vi "Teleop.vi"(10 "Match Info":T1={"Autonomous Elapsed Seconds"=0.0, "TeleOp Elapsed Seconds"=0.0, "Disabled Elapsed Seconds"=0.0, "Visited Autonomous"=FALSE, "Visited TeleOp"=FALSE, "Visited Disabled"=FALSE, "Autonomous Settings"={"Autonomous Style"=enum."Independent", "VI Refnum"=refnum}}, 11 "Call Context":T2) -> ()   [LabVIEW 2017]
doc: "This VI is called for each enabled TeleOp packet received from the DS. It is typically used to read from joysticks and other inputs and update I/O or setpoints for timed control loops. It should complete and return within 20 milliseconds or risk missing DS packets."
uses:
  <vilib>/Rock Robotics/WPI/DriverStation/WPI_DriverStationDerivedRobotMode.ctl
  <vilib>/Rock Robotics/WPI/DriverStation/WPI_DriverStationMatch Info.ctl
  Framework/Robot Global Data.vi
panel:
  out "Hardware Fault":bool
  out "Temperature Fault":bool
  out "Battery Voltage Fault":bool
  out "Current Faults":bool[](array[boolean])
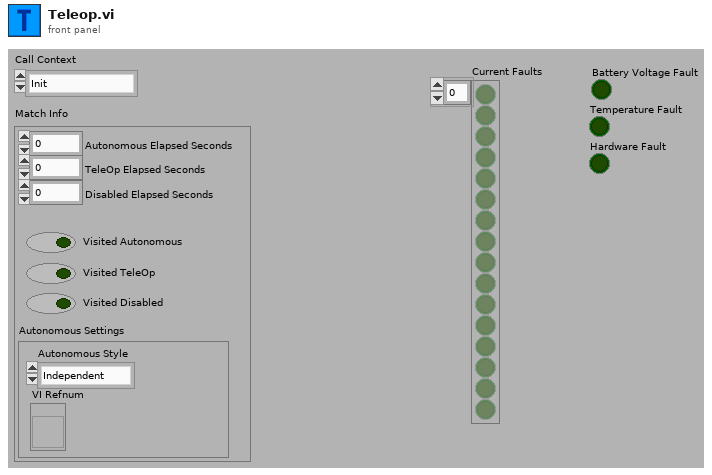
[diagram p1: front panel]
types:
  T1 = typedef "WPI_DriverStationMatch Info.ctl" = cluster{"Autonomous Elapsed Seconds":dbl, "TeleOp Elapsed Seconds":dbl, "Disabled Elapsed Seconds":dbl, "Visited Autonomous":bool, "Visited TeleOp":bool, "Visited Disabled":bool, "Autonomous Settings":cluster{"Autonomous Style":enum16{"Iterative", "Independent"}, "VI Refnum":refnum<vi>}}
  T2 = typedef "WPI_DriverStationDerivedRobotMode.ctl" = enum16{"Init", "Execute", "Stop"}
  T3 = enum16{"Linear", "Square  Root", "Square", "n^x"}
  T4 = enum16{"Normal", "Square", "Square with Rate", "Square Root", "Linear", "Exponential"}
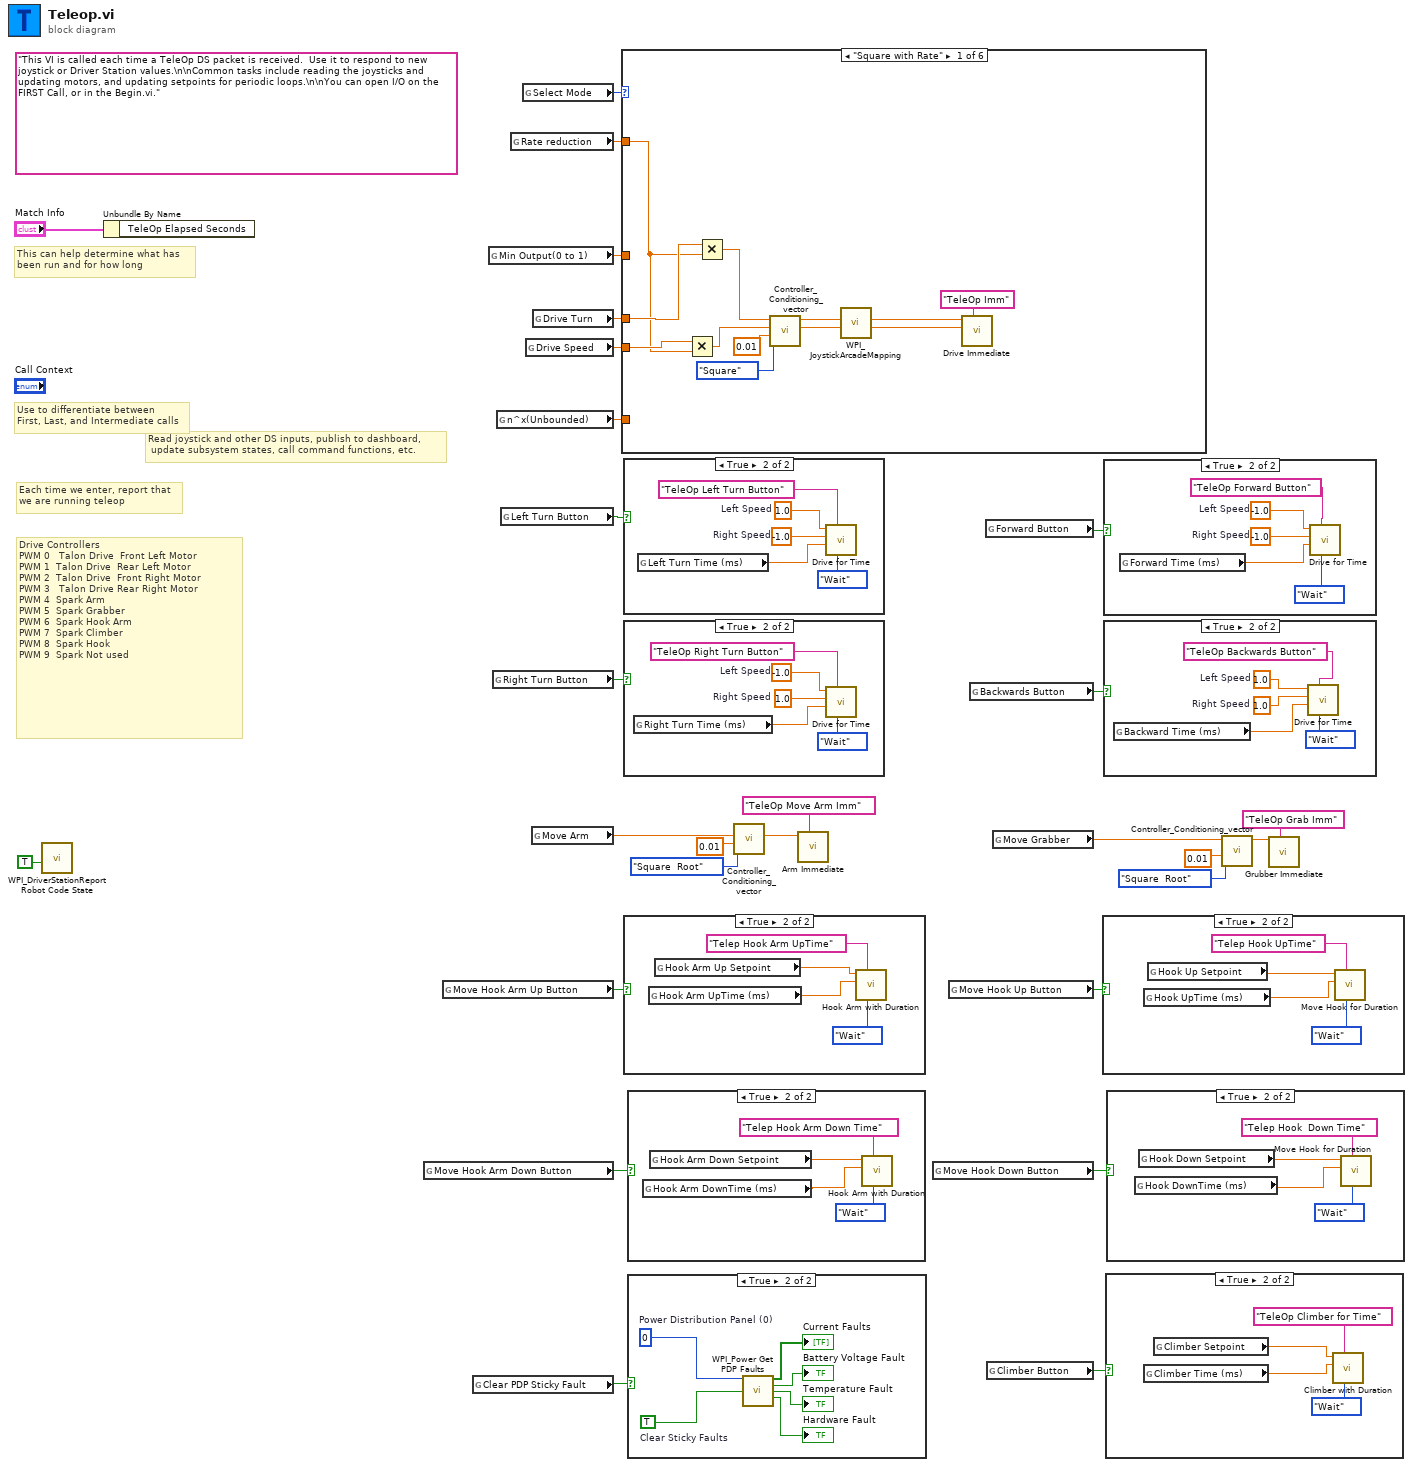
[diagram p0: block diagram]
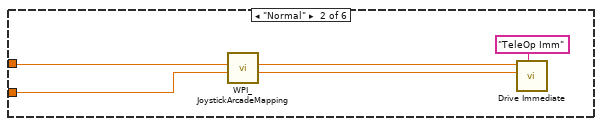
[diagram p12: hidden frame]
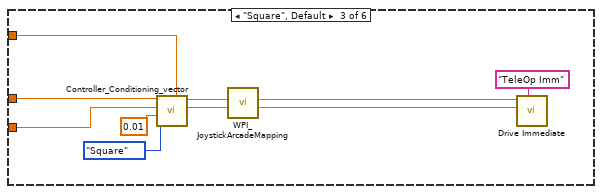
[diagram p13: hidden frame]
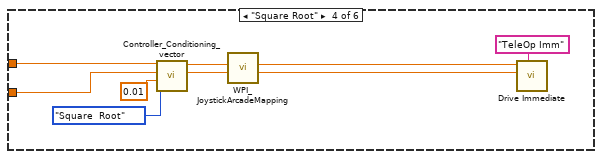
[diagram p14: hidden frame]
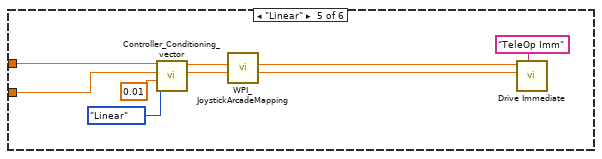
[diagram p15: hidden frame]
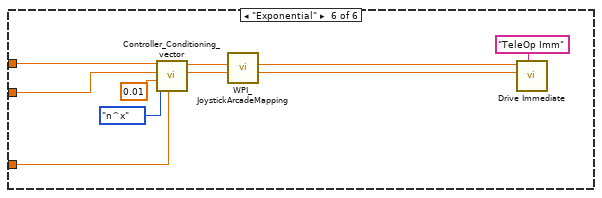
[diagram p16: hidden frame]
diagram:
  (unwired) "This VI is called each time a TeleOp DS packet is received.  Use it to respond to new joystick or Driver Station values.\n\nCommon tasks include reading the joysticks and updating motors, and updating setpoints for periodic loops.\n\nYou can open I/O on the FIRST Call, or in the Begin.vi."
  # "Drive Controllers\nPWM 0 \t\tTalon\tDrive \tFront Left Motor\nPWM 1\t\tTalon\tDrive \tRear Left Motor\nPWM 2\t\tTalon\tDrive \tFront Right Motor\nPWM 3 \t\tTalon\tDrive\tRear Right Motor\nPWM 4\t\tSpark\tArm\nPWM 5\t\tSpark\tGrabber\nPWM 6\t\tSpark\tHook Arm\nPWM 7\t\tSpark\tClimber\nPWM 8\t\tSpark\tHook\nPWM 9\t\tSpark\tNot used"
  # "Read joystick and other DS inputs, publish to dashboard,\n update subsystem states, call command functions, etc."
  # "Each time we enter, report that\nwe are running teleop"
  # "Use to differentiate between\nFirst, Last, and Intermediate calls"
  # "This can help determine what has\nbeen run and for how long"
  n1 = call <vilib>:"WPI_DriverStationReport Robot Code State.vi"("TeleOp"=TRUE ("Autonomous")) -> ()  [unwired: 10 in, 1 out]
  n2 = Unbundle By Name("Match Info") -> ()  [unwired: 1 out]
  n3 = global read "Robot Global Data.vi" "Move Hook Arm Down Button"() -> (w14:bool)
  n4 = global read "Robot Global Data.vi" "Move Hook Arm Up Button"() -> (w15:bool)
  n5 = global read "Robot Global Data.vi" "Clear PDP Sticky Fault"() -> (w16:bool)
  n6 = global read "Robot Global Data.vi" "Min Output(0 to 1)"() -> (w25:dbl)
  n7 = global read "Robot Global Data.vi" "Right Turn Button"() -> (w19:bool)
  n8 = global read "Robot Global Data.vi" "n^x(Unbounded)"() -> (w24:dbl)
  n9 = global read "Robot Global Data.vi" "Left Turn Button"() -> (w20:bool)
  n10 = global read "Robot Global Data.vi" "Rate reduction"() -> (w23:dbl)
  n11 = global read "Robot Global Data.vi" "Select Mode"() -> (w26:T4)
  n12 = global read "Robot Global Data.vi" "Drive Speed"() -> (w21:dbl)
  n13 = global read "Robot Global Data.vi" "Move Arm"() -> (w18:dbl)
  n14 = global read "Robot Global Data.vi" "Drive Turn"() -> (w22:dbl)
  n15 = case shown="\"Square with Rate\"" w26 {
    tunnel: w22 -> [w40 w42 w47 w56 w65 w75]
    tunnel: w21 -> [w39 w41 w48 w57 w66 w76]
    tunnel: w25 -> [_ _ w46 _ _ _]
    tunnel: w24 -> [_ _ _ _ _ w74]
    tunnel: w23 -> [w29 _ _ _ _ _]
    frame "Square with Rate" {
      n16 = Multiply(x=w39, y=w29) -> (x*y=w30:dbl)
      n17 = Multiply(x=w40, y=w29) -> (x*y=w31:dbl)
      n18 = call "Controller_Conditioning_vector.vi"("Enum"=T3."Square", "Dead Zone(0 to 1)"=0.01, "Y(-1 to 1)"=w30, "X(-1 to 1)"=w31) -> ("Y"=w32:dbl, "X"=w33:dbl)  [unwired: 4 in, 2 out]
      n19 = call <vilib>:"WPI_JoystickArcadeMapping.vi"("Y axis value"=w32, "X axis value"=w33) -> ("Right Motor Value"=w36:dbl, "Left Motor Value"=w37:dbl)  [unwired: 8 in]
      n20 = call "Drive Immediate.vi"("Description"="TeleOp Imm", "Right Setpoint"=w36, "Left Setpoint"=w37) -> ()  [unwired: 8 in, 1 out]
    }
    frame "Normal" {
      n21 = call <vilib>:"WPI_JoystickArcadeMapping.vi"("Y axis value"=w41, "X axis value"=w42) -> ("Right Motor Value"=w43:dbl, "Left Motor Value"=w44:dbl)  [unwired: 8 in]
      n22 = call "Drive Immediate.vi"("Description"="TeleOp Imm", "Right Setpoint"=w43, "Left Setpoint"=w44) -> ()  [unwired: 8 in, 1 out]
    }
    frame "Square", Default {
      n23 = call "Controller_Conditioning_vector.vi"("Min Output(0 to 1)"=w46, "Enum"=T3."Square", "Dead Zone(0 to 1)"=0.01, "Y(-1 to 1)"=w48, "X(-1 to 1)"=w47) -> ("Y"=w49:dbl, "X"=w50:dbl)  [unwired: 3 in, 2 out]
      n24 = call <vilib>:"WPI_JoystickArcadeMapping.vi"("Y axis value"=w49, "X axis value"=w50) -> ("Right Motor Value"=w53:dbl, "Left Motor Value"=w54:dbl)  [unwired: 8 in]
      n25 = call "Drive Immediate.vi"("Description"="TeleOp Imm", "Right Setpoint"=w53, "Left Setpoint"=w54) -> ()  [unwired: 8 in, 1 out]
    }
    frame "Square Root" {
      n26 = call "Controller_Conditioning_vector.vi"("Enum"=T3."Square  Root", "Dead Zone(0 to 1)"=0.01, "Y(-1 to 1)"=w57, "X(-1 to 1)"=w56) -> ("Y"=w58:dbl, "X"=w59:dbl)  [unwired: 4 in, 2 out]
      n27 = call <vilib>:"WPI_JoystickArcadeMapping.vi"("Y axis value"=w58, "X axis value"=w59) -> ("Right Motor Value"=w62:dbl, "Left Motor Value"=w63:dbl)  [unwired: 8 in]
      n28 = call "Drive Immediate.vi"("Description"="TeleOp Imm", "Right Setpoint"=w62, "Left Setpoint"=w63) -> ()  [unwired: 8 in, 1 out]
    }
    frame "Linear" {
      n29 = call "Controller_Conditioning_vector.vi"("Enum"=T3."Linear", "Dead Zone(0 to 1)"=0.01, "Y(-1 to 1)"=w66, "X(-1 to 1)"=w65) -> ("Y"=w67:dbl, "X"=w68:dbl)  [unwired: 4 in, 2 out]
      n30 = call <vilib>:"WPI_JoystickArcadeMapping.vi"("Y axis value"=w67, "X axis value"=w68) -> ("Right Motor Value"=w71:dbl, "Left Motor Value"=w72:dbl)  [unwired: 8 in]
      n31 = call "Drive Immediate.vi"("Description"="TeleOp Imm", "Right Setpoint"=w71, "Left Setpoint"=w72) -> ()  [unwired: 8 in, 1 out]
    }
    frame "Exponential" {
      n32 = call "Controller_Conditioning_vector.vi"("n^x(Unbounded)"=w74, "Enum"=T3."n^x", "Dead Zone(0 to 1)"=0.01, "Y(-1 to 1)"=w76, "X(-1 to 1)"=w75) -> ("Y"=w77:dbl, "X"=w78:dbl)  [unwired: 3 in, 2 out]
      n33 = call <vilib>:"WPI_JoystickArcadeMapping.vi"("Y axis value"=w77, "X axis value"=w78) -> ("Right Motor Value"=w81:dbl, "Left Motor Value"=w82:dbl)  [unwired: 8 in]
      n34 = call "Drive Immediate.vi"("Description"="TeleOp Imm", "Right Setpoint"=w81, "Left Setpoint"=w82) -> ()  [unwired: 8 in, 1 out]
    }
  }
  n35 = case shown="True" w20 {
    frame False {
    }
    frame True {
      w86 = -1.0  # Right Speed
      w85 = 1.0  # Left Speed
      n36 = global read "Robot Global Data.vi" "Left Turn Time (ms)"() -> (w84:dbl)
      n37 = call "Drive for Time.vi"("Synchronization"=enum16{"Start", "Wait"}."Wait" ("Synchronication"), "Description"="TeleOp Left Turn Button", "Duration (ms)"=w84, "Right Speed"=w86, "Left Speed"=w85) -> ()  [unwired: 5 in, 2 out]
    }
  }
  n38 = case shown="True" w19 {
    frame False {
    }
    frame True {
      w91 = 1.0  # Right Speed
      w90 = -1.0  # Left Speed
      n39 = global read "Robot Global Data.vi" "Right Turn Time (ms)"() -> (w89:dbl)
      n40 = call "Drive for Time.vi"("Synchronization"=enum16{"Start", "Wait"}."Wait" ("Synchronication"), "Description"="TeleOp Right Turn Button", "Duration (ms)"=w89, "Right Speed"=w91, "Left Speed"=w90) -> ()  [unwired: 5 in, 2 out]
    }
  }
  n41 = case shown="True" w15 {
    frame False {
    }
    frame True {
      n42 = global read "Robot Global Data.vi" "Hook Arm UpTime (ms)"() -> (w95:dbl)
      n43 = global read "Robot Global Data.vi" "Hook Arm Up Setpoint"() -> (w94:dbl)
      n44 = call "Hook Arm with Duration.vi"("Synchronization"=enum16{"Start", "Wait"}."Wait", "Description"="Telep Hook Arm UpTime", "Duration (ms)"=w95, "Setpoint"=w94) -> ()  [unwired: 7 in, 1 out]
    }
  }
  n45 = case shown="True" w14 {
    frame False {
    }
    frame True {
      n46 = global read "Robot Global Data.vi" "Hook Arm DownTime (ms)"() -> (w99:dbl)
      n47 = global read "Robot Global Data.vi" "Hook Arm Down Setpoint"() -> (w98:dbl)
      n48 = call "Hook Arm with Duration.vi"("Synchronization"=enum16{"Start", "Wait"}."Wait", "Description"="Telep Hook Arm Down Time", "Duration (ms)"=w99, "Setpoint"=w98) -> ()  [unwired: 7 in, 1 out]
    }
  }
  n49 = case shown="True" w16 {
    frame False {
    }
    frame True {
      w106 = TRUE  # Clear Sticky Faults
      w107 = u8 0  # Power Distribution Panel (0)
      n50 = call <vilib>:"WPI_Power Get PDP Faults.vi"("Power Distribution Panel (0)"=w107, "Clear Sticky Faults"=w106) -> ("Current Faults"=→"Current Faults":bool[], "Battery Voltage Fault"=→"Battery Voltage Fault":bool, "Temperature Fault"=→"Temperature Fault":bool, "Hardware Fault"=→"Hardware Fault":bool)  [unwired: 9 in, 1 out]
    }
  }
  n51 = call "Controller_Conditioning_vector.vi"("Enum"=T3."Square  Root", "Dead Zone(0 to 1)"=0.01, "Y(-1 to 1)"=w18) -> ("Y"=w9:dbl)  [unwired: 5 in, 3 out]
  n52 = call "Arm Immediate.vi"("Description"="TeleOp Move Arm Imm", "Setpoint"=w9) -> ()  [unwired: 9 in, 1 out]
  n53 = global read "Robot Global Data.vi" "Move Hook Down Button"() -> (w3:bool)
  n54 = global read "Robot Global Data.vi" "Move Hook Up Button"() -> (w2:bool)
  n55 = global read "Robot Global Data.vi" "Backwards Button"() -> (w13:bool)
  n56 = global read "Robot Global Data.vi" "Forward Button"() -> (w12:bool)
  n57 = global read "Robot Global Data.vi" "Climber Button"() -> (w1:bool)
  n58 = global read "Robot Global Data.vi" "Move Grabber"() -> (w17:dbl)
  n59 = case shown="True" w2 {
    frame False {
    }
    frame True {
      n60 = global read "Robot Global Data.vi" "Hook UpTime (ms)"() -> (w109:dbl)
      n61 = global read "Robot Global Data.vi" "Hook Up Setpoint"() -> (w108:dbl)
      n62 = call "Move Hook for Duration.vi"("Synchronization"=enum16{"Start", "Wait"}."Wait", "Description"="Telep Hook UpTime", "Duration (ms)"=w109, "Setpoint"=w108) -> ()  [unwired: 7 in, 1 out]
    }
  }
  n63 = case shown="True" w12 {
    frame False {
    }
    frame True {
      w113 = -1.0  # Right Speed
      w114 = -1.0  # Left Speed
      n64 = global read "Robot Global Data.vi" "Forward Time (ms)"() -> (w112:dbl)
      n65 = call "Drive for Time.vi"("Synchronization"=enum16{"Start", "Wait"}."Wait", "Description"="TeleOp Forward Button", "Duration (ms)"=w112, "Right Speed"=w113, "Left Speed"=w114) -> ()  [unwired: 5 in, 2 out]
    }
  }
  n66 = case shown="True" w13 {
    frame False {
    }
    frame True {
      w118 = 1.0  # Right Speed
      w119 = 1.0  # Left Speed
      n67 = global read "Robot Global Data.vi" "Backward Time (ms)"() -> (w117:dbl)
      n68 = call "Drive for Time.vi"("Synchronization"=enum16{"Start", "Wait"}."Wait", "Description"="TeleOp Backwards Button", "Duration (ms)"=w117, "Right Speed"=w118, "Left Speed"=w119) -> ()  [unwired: 5 in, 2 out]
    }
  }
  n69 = case shown="True" w1 {
    frame False {
    }
    frame True {
      n70 = global read "Robot Global Data.vi" "Climber Time (ms)"() -> (w122:dbl)
      n71 = global read "Robot Global Data.vi" "Climber Setpoint"() -> (w123:dbl)
      n72 = call "Climber with Duration.vi"("Synchronization"=enum16{"Start", "Wait"}."Wait", "Description"="TeleOp Climber for Time", "Duration (ms)"=w122, "Setpoint"=w123) -> ()  [unwired: 7 in, 1 out]
    }
  }
  n73 = case shown="True" w3 {
    frame False {
    }
    frame True {
      n74 = global read "Robot Global Data.vi" "Hook DownTime (ms)"() -> (w127:dbl)
      n75 = global read "Robot Global Data.vi" "Hook Down Setpoint"() -> (w126:dbl)
      n76 = call "Move Hook for Duration.vi"("Synchronization"=enum16{"Start", "Wait"}."Wait", "Description"="Telep Hook  Down Time", "Duration (ms)"=w127, "Setpoint"=w126) -> ()  [unwired: 7 in, 1 out]
    }
  }
  n77 = call "Controller_Conditioning_vector.vi"("Enum"=T3."Square  Root", "Dead Zone(0 to 1)"=0.01, "X(-1 to 1)"=w17) -> ("X"=w6:dbl)  [unwired: 5 in, 3 out]
  n78 = call "Grubber Immediate.vi"("Description"="TeleOp Grab Imm", "Setpoint"=w6) -> ()  [unwired: 9 in, 1 out]
